vi "Event Handle Loop_Drag Panel.vi"(8 "error in (no error)":errorcluster, 11 "QTab Class in":refnum<class "QTab Class.lvclass">) -> (0 "error out":errorcluster, 2 "Confirm":bool, 3 "QTab Class out":refnum<class "QTab Class.lvclass">)   [LabVIEW 2020, in "QTab.lvlib" / "QTab Class.lvclass"]
uses:
  QTab Class.lvclass
  QTab Class.lvclass/QTab Class.ctl
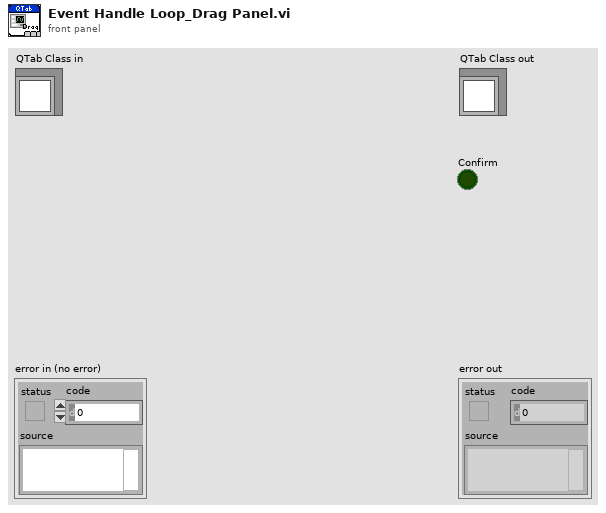
[diagram p1: front panel]
types:
  T1 = typedef "QTab.lvlib/QTab Class.lvclass/Pag Attribute.ctl" = cluster{"VI Refnum":refnum<vi>, "Page Name":string, "Closeable":bool, "Draggable":bool, "Pop-Out":bool}
  T2 = typedef "LVRectTypeDef.ctl" = cluster{"Left":i16, "Top":i16, "Right":i16, "Bottom":i16}
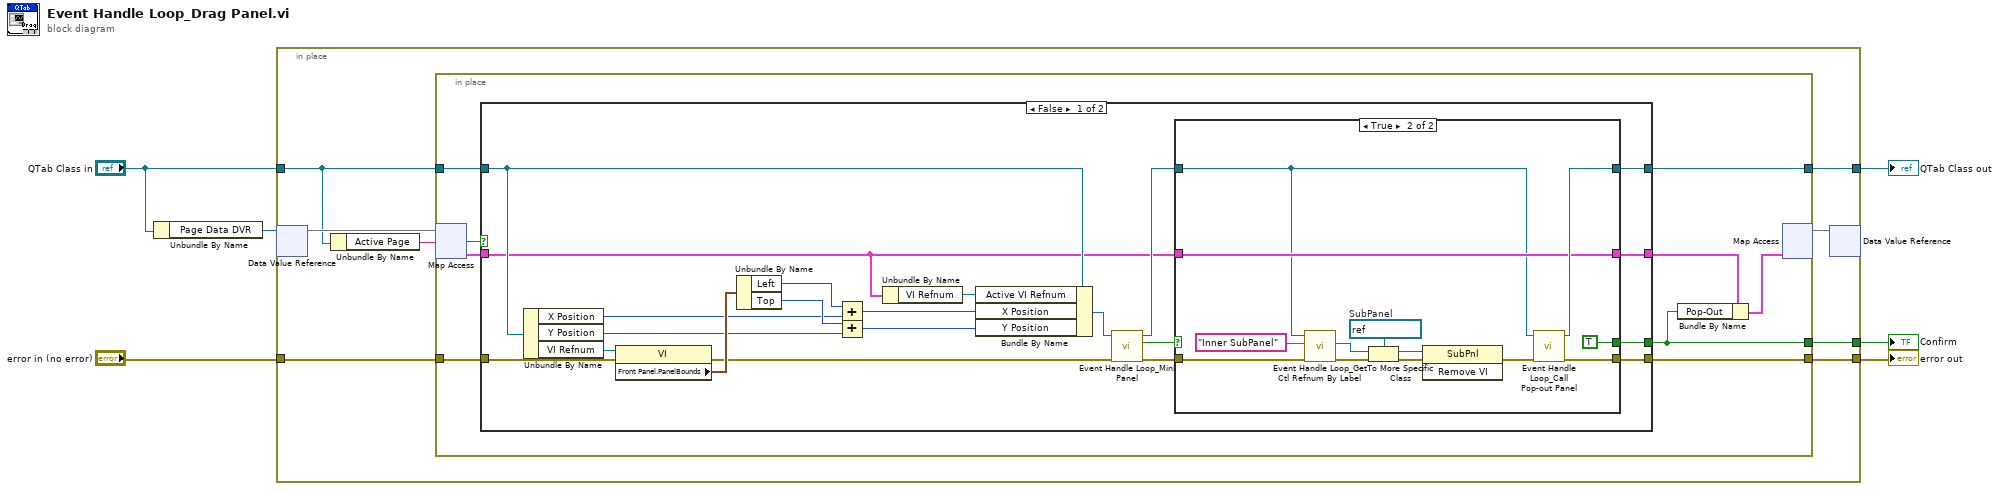
[diagram p0: block diagram]
diagram:
  n1 = Unbundle By Name("QTab Class in") -> ("Page Data DVR"=w1:refnum<data-value>)
  n2 = in-place {
    in-place-border: "error in (no error)" -> [w14]
    in-place-border: "QTab Class in" -> [w9]
    in-place-border: [w13] -> w4
    in-place-border: [w12] -> w3
    in-place-border: [w11] -> w2
    n3 = in-place-dvr #1(w1) -> (w10:map{string, T1})  [unwired: 1 out]
    n4 = Unbundle By Name(w9) -> ("Active Page"=w8:string)
    n5 = in-place {
      in-place-border: w14 -> [w23]
      in-place-border: w9 -> [w22]
      in-place-border: [w21] -> w13
      in-place-border: [w20] -> w12
      in-place-border: [w16] -> w11
      n6 = in-place-map #2(w10, w8) -> (w18:T1, w19:bool)  [unwired: 1 in]
      n7 = case shown="False" w19 {
        tunnel: w23 -> [w44 w62]
        tunnel: [w32 w62] -> w20
        tunnel: w22 -> [w37 w63]
        tunnel: [w33 w63] -> w21
        tunnel: [w31 _] -> w16
        tunnel: w18 -> [w26 w61]
        tunnel: [w24 w61] -> w17
        frame False {
          n8 = Unbundle By Name(w37) -> ("X Position"=w28:i16, "Y Position"=w27:i16, "VI Refnum"=w43:refnum<vi>)
          n9 = property class="VI"(reference=w43, error in=w44) -> (error out=w39:errorcluster, "Front Panel.PanelBounds"=w41:T2)  [unwired: 1 out]
          n10 = Unbundle By Name(w41) -> ("Left"=w42:i16, "Top"=w40:i16)
          n11 = Add(x=w42, y=w28) -> (x+y=w30:i16)
          n12 = Add(x=w40, y=w27) -> (x+y=w29:i16)
          n13 = Unbundle By Name(w26) -> ("VI Refnum"=w25:refnum<vi>)
          n14 = Bundle By Name(cluster=w37, "Active VI Refnum"=w25, "X Position"=w30, "Y Position"=w29) -> (w38:refnum<class "QTab Class.lvclass">)
          n15 = call "Event Handle Loop_Mini Panel.vi"("error in (no error)"=w39, "QTab Class in"=w38) -> ("error out"=w36:errorcluster, "OK?"=w35:bool, "QTab Class Out"=w34:refnum<class "QTab Class.lvclass">)  [unwired: 7 in]
          n16 = case shown="True" w35 {
            tunnel: w36 -> [w46 w51]
            tunnel: w34 -> [w47 w49]
            tunnel: [w47 w60] -> w33
            tunnel: [w46 w59] -> w32
            tunnel: [_ TRUE] -> w31
            tunnel: w26 -> [w45 w58]
            tunnel: [w45 w58] -> w24
            frame False {
            }
            frame True {
              w53 = refnum<vi> refnum  # SubPanel
              n17 = call "Event Handle Loop_Get Ctl Refnum By Label.vi"("error in (no error)"=w51, "Label"="Inner SubPanel", "QTab Class in"=w49) -> ("error out"=w55:errorcluster, "Ctl Refnum"=w54:refnum<vi>)  [unwired: 6 in, 1 out]
              n18 = To More Specific Class(target class=w53, reference=w54, error in=w55) -> (specific class reference=w56:refnum<vi>, error out=w57:errorcluster)
              n19 = invoke class="SubPnl" method="Remove VI"(reference=w56, error in=w57) -> (error out=w50:errorcluster)  [unwired: 1 in, 2 out]
              n20 = call "Event Handle Loop_Call Pop-out Panel.vi"("error in (no error)"=w50, "QTab Class in"=w49) -> ("error out"=w59:errorcluster, "QTab Class out"=w60:refnum<class "QTab Class.lvclass">)  [unwired: 8 in]
            }
          }
        }
        frame True {
        }
      }
      n21 = Bundle By Name(cluster=w17, "Pop-Out"=w16) -> (w15:T1)
      n22 = in-place-map #2(w15) -> (w7:map{string, T1})  [unwired: 1 in, 2 out]
    }
    n23 = in-place-dvr #1(w7) -> ()  [unwired: 2 out]
  }
  "error out" <- w3
  "QTab Class out" <- w4
  "Confirm" <- w2
